vi "CAPTH-Insert Notes.vi"(0 "path":path, 7 "Notes":string, 11 "error in (no error)":errorcluster) -> (15 "error out":errorcluster)   [LabVIEW 2020]
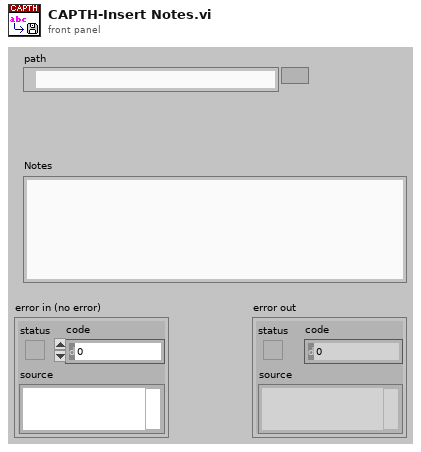
[diagram p1: front panel]
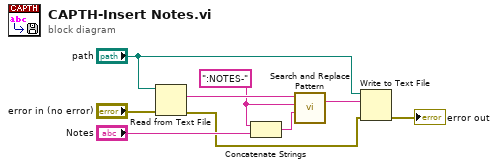
[diagram p0: block diagram]
diagram:
  w8 = ":NOTES-" ("regular expression (\"\")")
  n1 = Read from Text File(file (use dialog)="path", error in="error in (no error)") -> (text=w9:string, error out=w3:errorcluster)  [unwired: 2 in, 2 out]
  n2 = Concatenate Strings(w8, "Notes") -> (w6:string)
  n3 = call <vilib>:"Search and Replace Pattern.vi"("string"=w9, "regular expression (\"\")"=w8, "replace string (\"\")"=w6) -> ("result string"=w4:string)  [unwired: 2 in, 1 out]
  n4 = Write to Text File(file (use dialog)="path", text=w4, error in=w3) -> (error out=→"error out":errorcluster)  [unwired: 1 in, 2 out]
